vi "Event Receive.vi"(11 "Base Event jettl in":refnum<class "Base Event jettl.lvclass">) -> (2 "Msg Strategy Event Registration":refnum<event-registration>, 3 "Base Event jettl out":refnum<class "Base Event jettl.lvclass">)   [LabVIEW 2021, in "jettl.lvlib" / "Base Event jettl.lvlib" / "Base Event jettl.lvclass"]
uses:
  Base Event jettl.lvclass
  Msg Strategy/Msg Strategy.lvclass
  Base Event jettl.lvclass/Base Event jettl.ctl
  jettl.lvlib
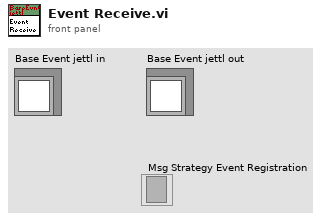
[diagram p1: front panel]
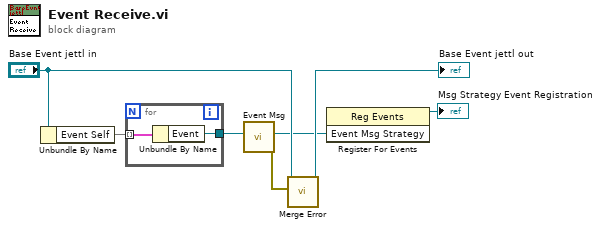
[diagram p0: block diagram]
diagram:
  n1 = Unbundle By Name("Base Event jettl in") -> ("Event Self"=w5:map{string, refnum<data-value>})
  n2 = for {
    tunnel: w5 -> [w9] mode=indexing
    tunnel: [w8] -> w4
    n3 = Unbundle By Name(w9) -> ("Event"=w8:refnum<data-value>)
  }
  n4 = call "Event Msg.vi"("Event"=w4) -> ("error out"=w3:errorcluster, "Event Msg Strategy"=w2:refnum<user-event>)  [unwired: 9 in]
  n5 = call-dynamic "Merge Error.vi"("Error"=w3, "Base Event jettl in"="Base Event jettl in") -> ("Base Event jettl out"=→"Base Event jettl out":refnum<class "Base Event jettl.lvclass">)  [unwired: 9 in]
  n6 = register-events(w2) -> (reference out=→"Msg Strategy Event Registration":refnum<event-registration>)  [unwired: 2 in, 1 out]
